vi "SPARC4_GUI.vi"() -> ()   [LabVIEW 2018]
uses:
  SPARC4_GUI/SPARC4_GUI.lvclass
  SPARC4_GUI/SPARC4_GUI.lvclass/SPARC4_GUI.ctl
  Channel GUI/Channel GUI.lvclass/Channel GUI.ctl
  Stream/Stream.lvclass/Stream.ctl
  Interface/Interface.lvclass/Interface.ctl
  Channel GUI/Channel GUI.lvclass
  Stream/Stream.lvclass
  State Machine/State Machine.lvclass
  Interface/Interface.lvclass
panel:
  out "Error":string
  in  "Tab Control 2":enum32{"Front Panel", "Setup Panel"}(tab)
  out "CCD Status":string
  out "Current image":string="CH1"
  out "% Acquired":u16
  out "Exposing":bool
  out "Temperature 2":i16
  out "Serial Number":u16
  out "Temperature Status":string
  in  "Base Name":string="IMG"
  in  "Exp Time 2":sgl=1e-05 min=1e-05
  in  "# Cubos":u32=1 min=1
  out "Exposições realizadas":u8(slide) max=2 scale=0.0..1.0
  in  "Acquire":bool
  in  "Command:":string
  out "Response:":string
  out "Initialization":bool
  in  "SEND":bool
  in  "IP Address:":string="//localhost"
  in  "Night Directory:":string="C:\\Users\\observer\\Desktop\\Imagens\\"
  in  "Stop Application":bool
  in  "Shutter Mode":u8(ring)=2 items=["Fully Auto", "OPEN", "CLOSED"]
  in  "Kinetic Series Length":u16=1 min=1
  in  "Cooler ON/OFF":u16(ring) items=["Cooler OFF", "Cooler ON"]
  in  "Temperature":i16=20 min=-80 max=20
  in  "Exposure Time":sgl=1e-05 min=1e-05
  in  "Readout Rate":u8(ring) items=["30 MHz", "20 MHz", "10 MHz", "  1 MHz"]
  in  "Pre-amp gain":u8(ring) items=["Gain 1", "Gain 2"]
  in  "EM Gain":u16=2
  in  "EM Mode":u8(ring) items=["Electron Multiplying", "Conventional"]
  in  "Sub Image":T1(radio)=enum."1024 x 1024"
  in  "Final Line":u16=1024
  in  "Final Column":u16=1024
  in  "Initial Cloumn":u16=1
  in  "Initial Line":u16=1
  in  "Binning":u16=1
  # "SPARC4 \nGeneral User Interface (GUI)"
  # "Command Acquisition Control"
  # "Channel 1: acquisition control & status"
  # "Temperature & Shutter"
  # "Timings"
  # "Horizontal pixel shift"
  # "EM Mode"
  # "Sub Image & Binning"
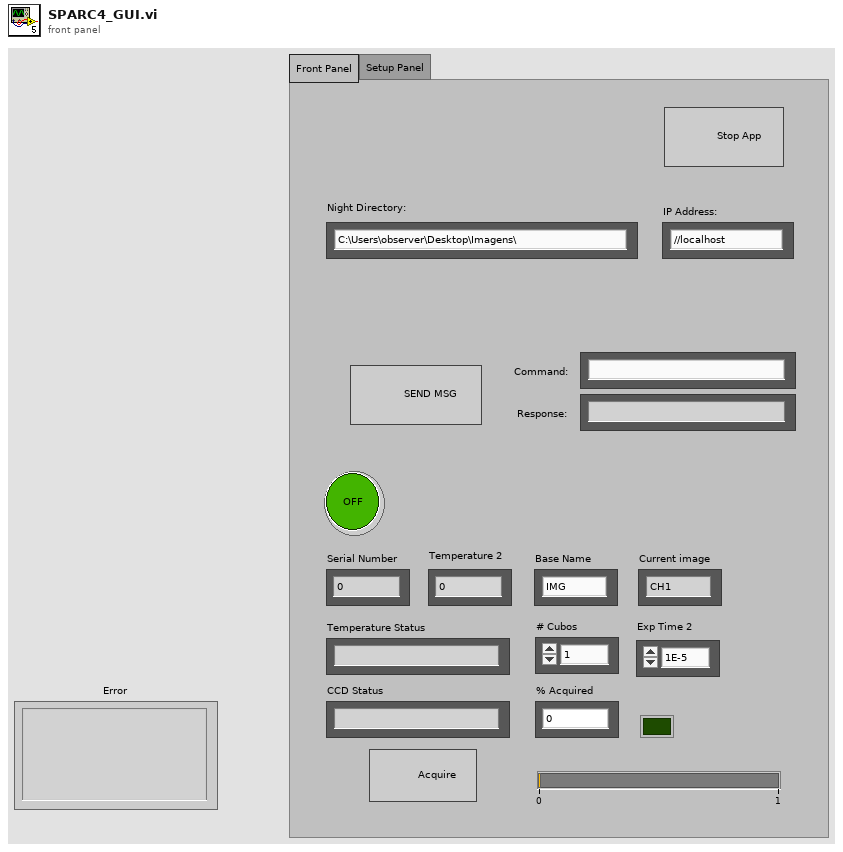
[diagram p1: front panel]
types:
  T1 = enum32{"256 x 256", "512 x 512", "1024 x 1024", "Custom"}
  T2 = cluster{"Exposure Time":sgl, "Pre-amp gain":u8, "Readout Rate":u8, "EM Mode":u8, "EM Gain":u16, "Binning":u16, "Initial Line":u16, "Initial Cloumn":u16, "Final Line":u16, "Final Column":u16, "Kinetic Series Length":u32, "Shutter Mode":u8, "Cooler ON/OFF":u16, "Temperature":i8, "Image Name":string, "Image Path":string, "# Images":u32}
  T3 = cluster{"% Acquired":u16, "Acquiring":bool, "Current image name":string, "Current sequence":u16, "CCD State":string}
  T4 = cluster{"Initialization":bool, "Serial Number":u16}
  T5 = cluster{"Current Temperature":i16, "Temperatue Status":string}
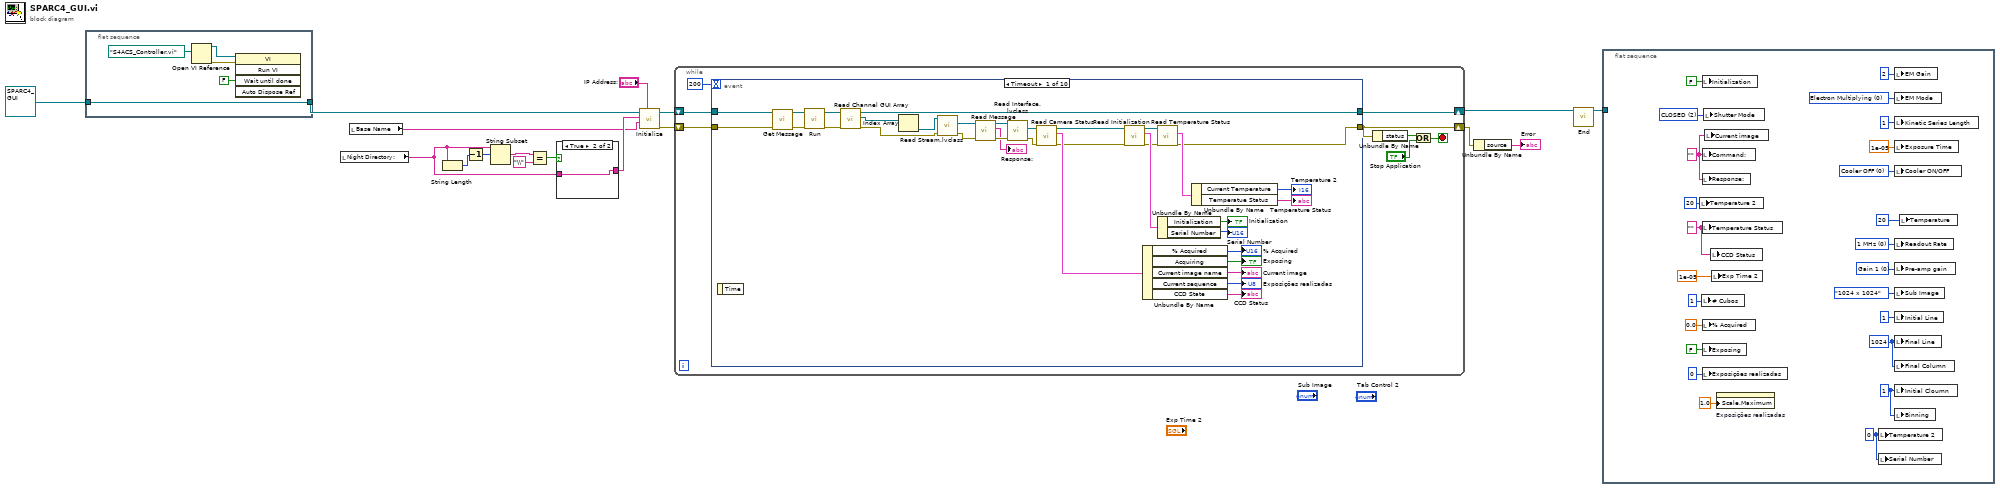
[diagram p0: block diagram]
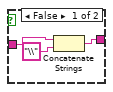
[diagram p2: hidden frame]
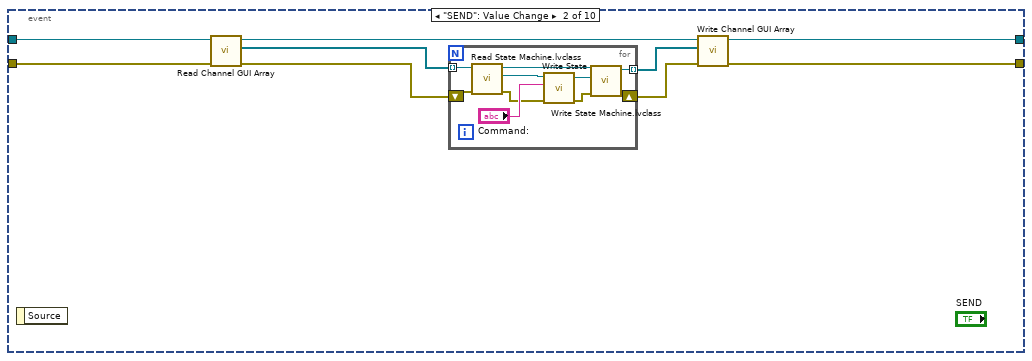
[diagram p3: hidden frame]
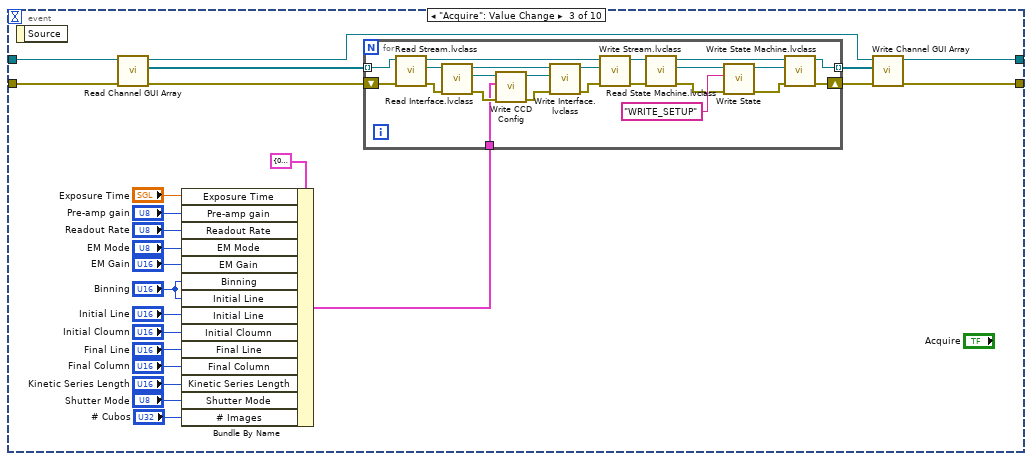
[diagram p4: hidden frame]
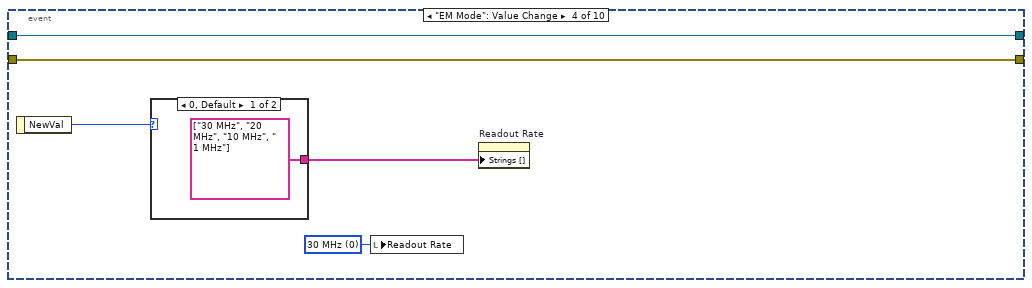
[diagram p5: hidden frame]
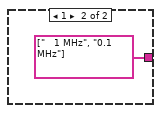
[diagram p6: hidden frame]
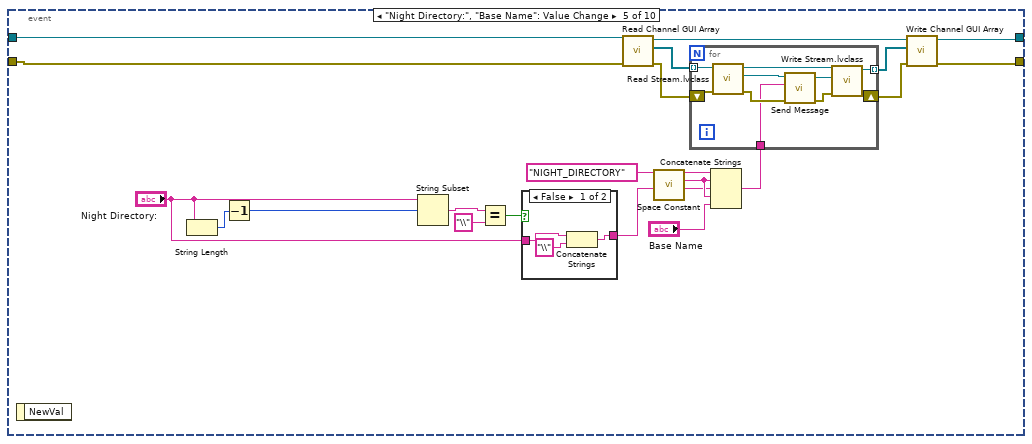
[diagram p7: hidden frame]
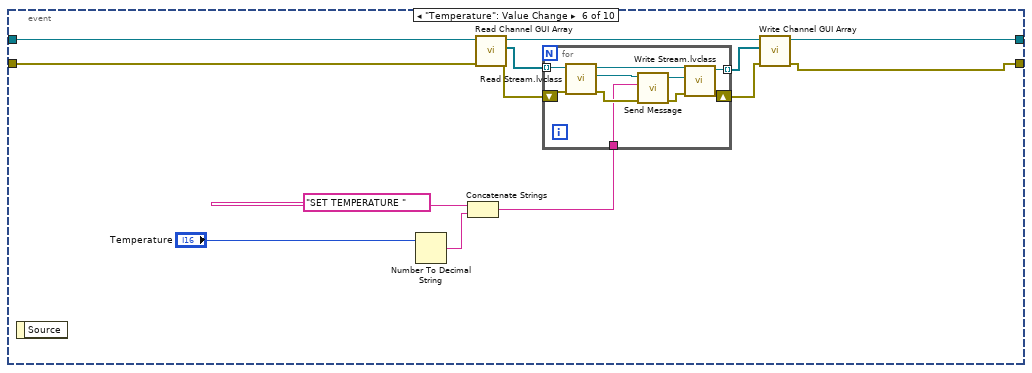
[diagram p9: hidden frame]
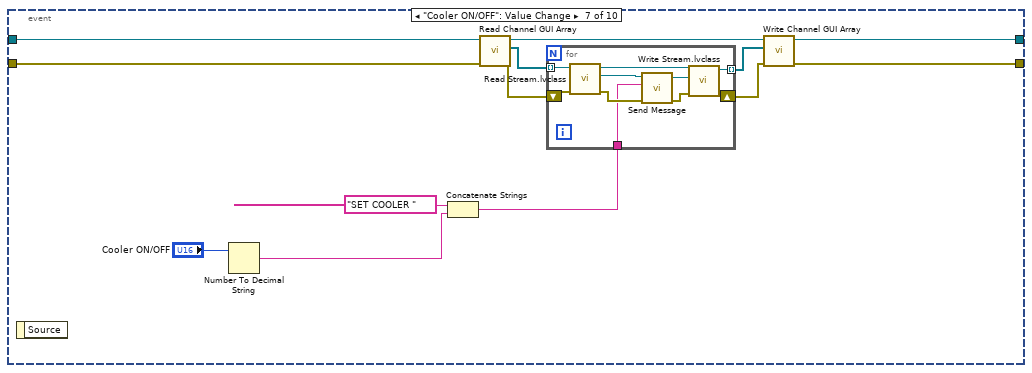
[diagram p10: hidden frame]
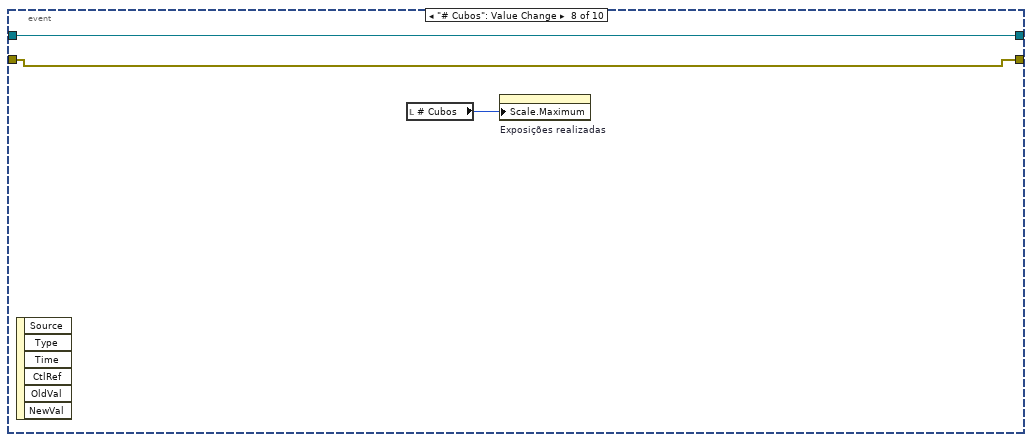
[diagram p11: hidden frame]
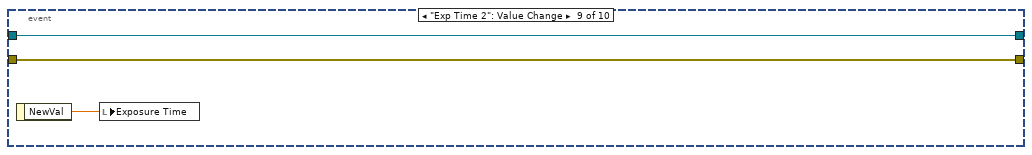
[diagram p12: hidden frame]
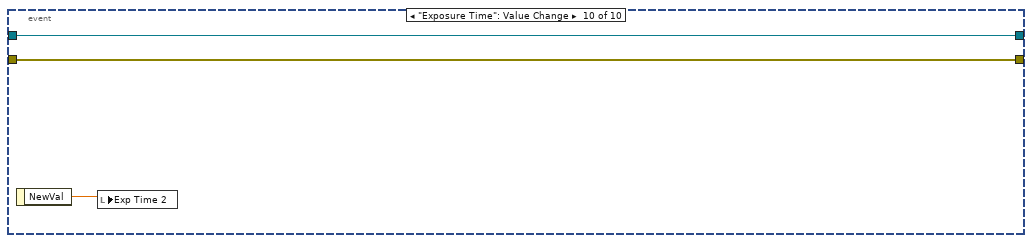
[diagram p13: hidden frame]
diagram:
  n1 = flat-sequence {
    tunnel: refnum<class "SPARC4_GUI.lvclass"> refnum ("SPARC4_GUI.lvclass") -> [w18]
    tunnel: [w18] -> w15
    frame #0 {
      n2 = Open VI Reference(vi path=path "S4ACS_Controller.vi") -> (vi reference=w22:refnum<vi>, error out=w21:errorcluster)  [unwired: 5 in]
      n3 = invoke class="VI" method="Run VI"(reference=w22, error in=w21, "Wait until done"=FALSE ("Wait Until Done")) -> ()  [unwired: 2 in, 5 out]
    }
  }
  n4 = local read "Night Directory:"() -> (w3:string)
  n5 = local read "Base Name"() -> (w1:string)
  n6 = String Length(string=w3) -> (length=w7:i32)
  n7 = Decrement(x=w7) -> (x-1=w6:i32)
  n8 = String Subset(string=w3, offset (0)=w6) -> (substring=w5:string)  [unwired: 1 in]
  n9 = Equal?(x=w5, y="\\") -> (x = y?=w4:bool)
  n10 = case shown="True" w4 {
    tunnel: [w25 w26] -> w2
    tunnel: w3 -> [w23 w26]
    frame False {
      n11 = Concatenate Strings(w23, "\\") -> (w25:string)
    }
    frame True {
    }
  }
  n12 = call "Initialize.vi"("IP"="IP Address:", "Image Name"=w1, "Night Directory:"=w2, "SPARC4_GUI in"=w15) -> ("error out"=w17:errorcluster, "SPARC4_GUI out"=w16:refnum<class "SPARC4_GUI.lvclass">)  [unwired: 6 in]
  n13 = while {
    shift-right: [w27] -> w10
    shift-left: w17 -> [w28]
    shift-right: [w30] -> w11
    shift-left: w16 -> [w29]
    stop <- w33 stop-if-true
    n14 = event shown="[0] Timeout" {
      selector: _ -> [_ _ _ _ _ _ _ _ _ _]
      dyn-events: _ -> [_ _ _ _ _ _ _ _ _ _]
      timeout: 200 -> [_ _ _ _ _ _ _ _ _ _]
      tunnel: w28 -> [w58 w76 w98 w138 w144 w178 w202 w223 w226 w229]
      tunnel: [w46 w69 w96 w138 w150 w184 w200 w223 w226 w229] -> w27
      tunnel: w29 -> [w59 w77 w99 w139 w143 w177 w203 w224 w227 w228]
      tunnel: [w57 w70 w97 w139 w151 w185 w201 w224 w227 w228] -> w30
      event Timeout {
        n15 = event-data() -> ()  [unwired: 1 in, 1 out]
        n16 = call "Get Message.vi"("error in (no error)"=w58, "SPARC4_GUI in"=w59) -> ("error out"=w61:errorcluster, "SPARC4_GUI out"=w60:refnum<class "SPARC4_GUI.lvclass">)  [unwired: 8 in]
        n17 = call "Run.vi"("error in (no error)"=w61, "SPARC4_GUI in"=w60) -> ("error out"=w66:errorcluster, "SPARC4_GUI out"=w65:refnum<class "SPARC4_GUI.lvclass">)  [unwired: 8 in]
        n18 = call "Read Channel GUI Array.vi"("error in (no error)"=w66, "SPARC4_GUI in"=w65) -> ("error out"=w36:errorcluster, "Channel GUI Array"=w38:refnum<class "Channel GUI.lvclass">[], "SPARC4_GUI out"=w57:refnum<class "SPARC4_GUI.lvclass">)  [unwired: 7 in]
        n19 = Index Array(array=w38) -> (element=w37:refnum<class "Channel GUI.lvclass">)  [unwired: 1 in]
        n20 = call "Read Stream.lvclass.vi"("error in (no error)"=w36, "Channel GUI in"=w37) -> ("error out"=w35:errorcluster, "Stream.lvclass"=w39:refnum<class "Stream.lvclass">)  [unwired: 7 in, 1 out]
        n21 = call "Read Message.vi"("error in (no error)"=w35, "Stream in"=w39) -> ("error out"=w44:errorcluster, "Message"=→"Response:":string, "Stream out"=w45:refnum<class "Stream.lvclass">)  [unwired: 7 in]
        n22 = call "Read Interface.lvclass.vi"("error in (no error)"=w44, "Stream in"=w45) -> ("error out"=w63:errorcluster, "Interface.lvclass"=w64:refnum<class "Interface.lvclass">)  [unwired: 7 in, 1 out]
        n23 = call "Read Camera Status.vi"("error in (no error)"=w63, "Interface in"=w64) -> ("error out"=w56:errorcluster, "Camera Status"=w62:T3, "Interface out"=w55:refnum<class "Interface.lvclass">)  [unwired: 7 in]
        n24 = call "Read Initialization.vi"("error in (no error)"=w56, "Interface in"=w55) -> ("error out"=w51:errorcluster, "Initialization"=w54:T4, "Interface out"=w50:refnum<class "Interface.lvclass">)  [unwired: 7 in]
        n25 = Unbundle By Name(w62) -> ("% Acquired"=→"% Acquired":u16, "Acquiring"=→"Exposing":bool, "Current image name"=→"Current image":string, "Current sequence"=→"Exposições realizadas":u16, "CCD State"=→"CCD Status":string)
        n26 = call "Read Temperature Status.vi"("error in (no error)"=w51, "Interface in"=w50) -> ("error out"=w46:errorcluster, "Temperature Status"=w49:T5)  [unwired: 7 in, 1 out]
        n27 = Unbundle By Name(w54) -> ("Initialization"=→"Initialization":bool, "Serial Number"=→"Serial Number":u16)
        n28 = Unbundle By Name(w49) -> ("Current Temperature"=→"Temperature 2":i16, "Temperatue Status"=→"Temperature Status":string)
      }
      event "SEND": Value Change {
        n29 = event-data() -> ()  [unwired: 1 in, 1 out]
        n30 = call "Read Channel GUI Array.vi"("error in (no error)"=w76, "SPARC4_GUI in"=w77) -> ("error out"=w72:errorcluster, "Channel GUI Array"=w75:refnum<class "Channel GUI.lvclass">[], "SPARC4_GUI out"=w71:refnum<class "SPARC4_GUI.lvclass">)  [unwired: 7 in]
        n31 = for {
          tunnel: w75 -> [w85] mode=indexing
          tunnel: [w86] -> w74 mode=indexing
          shift-right: [w80] -> w73
          shift-left: w72 -> [w79]
          n32 = call "Read State Machine.lvclass.vi"("error in (no error)"=w79, "Channel GUI in"=w85) -> ("error out"=w82:errorcluster, "State Machine.lvclass"=w83:refnum<class "State Machine.lvclass">, "Channel GUI out"=w84:refnum<class "Channel GUI.lvclass">)  [unwired: 7 in]
          n33 = call-dynamic "Write State.vi"("error in (no error)"=w82, "State"="Command:", "State Machine in"=w83) -> ("error out"=w81:errorcluster, "State Machine out"=w78:refnum<class "State Machine.lvclass">)  [unwired: 7 in]
          n34 = call "Write State Machine.lvclass.vi"("error in (no error)"=w81, "State Machine.lvclass"=w78, "Channel GUI in"=w84) -> ("error out"=w80:errorcluster, "Channel GUI out"=w86:refnum<class "Channel GUI.lvclass">)  [unwired: 7 in]
        }
        n35 = call "Write Channel GUI Array.vi"("error in (no error)"=w73, "Channel GUI Array"=w74, "SPARC4_GUI in"=w71) -> ("error out"=w69:errorcluster, "SPARC4_GUI out"=w70:refnum<class "SPARC4_GUI.lvclass">)  [unwired: 7 in]
      }
      event "Acquire": Value Change {
        n36 = event-data() -> ()  [unwired: 1 in, 1 out]
        n37 = call "Read Channel GUI Array.vi"("error in (no error)"=w98, "SPARC4_GUI in"=w99) -> ("error out"=w91:errorcluster, "Channel GUI Array"=w92:refnum<class "Channel GUI.lvclass">[], "SPARC4_GUI out"=w88:refnum<class "SPARC4_GUI.lvclass">)  [unwired: 7 in]
        n38 = Bundle By Name(cluster=T2 {"Exposure Time"=0.0, "Pre-amp gain"=0, "Readout Rate"=0, "EM Mode"=0, "EM Gain"=2, "Binning"=1, "Initial Line"=1, "Initial Cloumn"=1, "Final Line"=1024, "Final Column"=1024, "Kinetic Series Length"=0, "Shutter Mode"=2, "Cooler ON/OFF"=0, "Temperature"=20, "Image Name"="", "Image Path"="", "# Images"=1} ("CCD Config"), "Exposure Time"="Exposure Time", "Pre-amp gain"="Pre-amp gain", "Readout Rate"="Readout Rate", "EM Mode"="EM Mode", "EM Gain"="EM Gain", "Binning"="Binning", "Initial Line"="Binning", "Initial Line"="Initial Line", "Initial Cloumn"="Initial Cloumn", "Final Line"="Final Line", "Final Column"="Final Column", "Kinetic Series Length"="Kinetic Series Length", "Shutter Mode"="Shutter Mode", "# Images"="# Cubos") -> (w111:T2)
        n39 = for {
          tunnel: w111 -> [w132]
          tunnel: w92 -> [w115] mode=indexing
          tunnel: [w113] -> w90 mode=indexing
          shift-right: [w112] -> w89
          shift-left: w91 -> [w114]
          n40 = call "Read Stream.lvclass.vi"("error in (no error)"=w114, "Channel GUI in"=w115) -> ("error out"=w126:errorcluster, "Stream.lvclass"=w127:refnum<class "Stream.lvclass">, "Channel GUI out"=w123:refnum<class "Channel GUI.lvclass">)  [unwired: 7 in]
          n41 = call "Read Interface.lvclass.vi"("error in (no error)"=w126, "Stream in"=w127) -> ("error out"=w133:errorcluster, "Interface.lvclass"=w134:refnum<class "Interface.lvclass">, "Stream out"=w131:refnum<class "Stream.lvclass">)  [unwired: 7 in]
          n42 = call "Write CCD Config.vi"("error in (no error)"=w133, "CCD Config"=w132, "Interface in"=w134) -> ("error out"=w129:errorcluster, "Interface out"=w128:refnum<class "Interface.lvclass">)  [unwired: 7 in]
          n43 = call "Write Interface.lvclass.vi"("error in (no error)"=w129, "Interface.lvclass"=w128, "Stream in"=w131) -> ("error out"=w125:errorcluster, "Stream out"=w124:refnum<class "Stream.lvclass">)  [unwired: 7 in]
          n44 = call "Write Stream.lvclass.vi"("error in (no error)"=w125, "Stream.lvclass"=w124, "Channel GUI in"=w123) -> ("error out"=w122:errorcluster, "Channel GUI out"=w121:refnum<class "Channel GUI.lvclass">)  [unwired: 7 in]
          n45 = call "Read State Machine.lvclass.vi"("error in (no error)"=w122, "Channel GUI in"=w121) -> ("error out"=w116:errorcluster, "State Machine.lvclass"=w119:refnum<class "State Machine.lvclass">, "Channel GUI out"=w120:refnum<class "Channel GUI.lvclass">)  [unwired: 7 in]
          n46 = call-dynamic "Write State.vi"("error in (no error)"=w116, "State"="WRITE_SETUP", "State Machine in"=w119) -> ("error out"=w117:errorcluster, "State Machine out"=w118:refnum<class "State Machine.lvclass">)  [unwired: 7 in]
          n47 = call "Write State Machine.lvclass.vi"("error in (no error)"=w117, "State Machine.lvclass"=w118, "Channel GUI in"=w120) -> ("error out"=w112:errorcluster, "Channel GUI out"=w113:refnum<class "Channel GUI.lvclass">)  [unwired: 7 in]
        }
        n48 = call "Write Channel GUI Array.vi"("error in (no error)"=w89, "Channel GUI Array"=w90, "SPARC4_GUI in"=w88) -> ("error out"=w96:errorcluster, "SPARC4_GUI out"=w97:refnum<class "SPARC4_GUI.lvclass">)  [unwired: 7 in]
      }
      event "EM Mode": Value Change {
        w135 = u8 0 items=["30 MHz", "20 MHz", "10 MHz", "1 MHz"] ("Readout Rate")
        n49 = event-data() -> ("NewVal"=w136:u8)  [unwired: 1 in]
        n50 = case shown="0, Default" w136 {
          tunnel: [string[] ["30 MHz", "20 MHz", "10 MHz", "  1 MHz"] string[] ["   1 MHz", "0.1 MHz"]] -> w137
          frame 0, Default {
          }
          frame 1 {
          }
        }
        n51 = local write "Readout Rate"(w135) -> ()
        n52 = property on="Readout Rate" class="Ring (strict)"("Strings []"=w137) -> ()  [unwired: 2 in, 2 out]
      }
      event "Night Directory:", "Base Name": Value Change {
        n53 = event-data() -> ()  [unwired: 1 in, 1 out]
        n54 = String Length(string="Night Directory:") -> (length=w154:i32)
        n55 = Decrement(x=w154) -> (x-1=w155:i32)
        n56 = String Subset(string="Night Directory:", offset (0)=w155) -> (substring=w156:string)  [unwired: 1 in]
        n57 = Equal?(x=w156, y="\\") -> (x = y?=w157:bool)
        n58 = case shown="False" w157 {
          tunnel: [w174 w175] -> w152
          tunnel: "Night Directory:" -> [w172 w175]
          frame False {
            n59 = Concatenate Strings(w172, "\\") -> (w174:string)
          }
          frame True {
          }
        }
        n60 = call "Read Channel GUI Array.vi"("error in (no error)"=w144, "SPARC4_GUI in"=w143) -> ("error out"=w145:errorcluster, "Channel GUI Array"=w148:refnum<class "Channel GUI.lvclass">[], "SPARC4_GUI out"=w149:refnum<class "SPARC4_GUI.lvclass">)  [unwired: 7 in]
        n61 = call <vilib>:"Space Constant.vi"() -> ("String"=w160:string)
        n62 = Concatenate Strings("NIGHT_DIRECTORY" ("Message"), w160, w152, w160, "Base Name") -> (w142:string)
        n63 = for {
          tunnel: w148 -> [w170] mode=indexing
          tunnel: [w171] -> w147 mode=indexing
          shift-right: [w165] -> w146
          shift-left: w145 -> [w164]
          tunnel: w142 -> [w162]
          n64 = call "Read Stream.lvclass.vi"("error in (no error)"=w164, "Channel GUI in"=w170) -> ("error out"=w167:errorcluster, "Stream.lvclass"=w168:refnum<class "Stream.lvclass">, "Channel GUI out"=w169:refnum<class "Channel GUI.lvclass">)  [unwired: 7 in]
          n65 = call "Send Message.vi"("error in (no error)"=w167, "Message"=w162, "Stream in"=w168) -> ("error out"=w166:errorcluster, "Stream out"=w163:refnum<class "Stream.lvclass">)  [unwired: 7 in]
          n66 = call "Write Stream.lvclass.vi"("error in (no error)"=w166, "Stream.lvclass"=w163, "Channel GUI in"=w169) -> ("error out"=w165:errorcluster, "Channel GUI out"=w171:refnum<class "Channel GUI.lvclass">)  [unwired: 7 in]
        }
        n67 = call "Write Channel GUI Array.vi"("error in (no error)"=w146, "Channel GUI Array"=w147, "SPARC4_GUI in"=w149) -> ("error out"=w150:errorcluster, "SPARC4_GUI out"=w151:refnum<class "SPARC4_GUI.lvclass">)  [unwired: 7 in]
      }
      event "Temperature": Value Change {
        n68 = event-data() -> ()  [unwired: 1 in, 1 out]
        n69 = Number To Decimal String(number="Temperature") -> (decimal integer string=w187:string)  [unwired: 1 in]
        n70 = Concatenate Strings("SET TEMPERATURE " ("Message"), w187) -> (w176:string)
        n71 = call "Read Channel GUI Array.vi"("error in (no error)"=w178, "SPARC4_GUI in"=w177) -> ("error out"=w179:errorcluster, "Channel GUI Array"=w180:refnum<class "Channel GUI.lvclass">[], "SPARC4_GUI out"=w181:refnum<class "SPARC4_GUI.lvclass">)  [unwired: 7 in]
        n72 = for {
          tunnel: w180 -> [w197] mode=indexing
          tunnel: [w198] -> w182 mode=indexing
          shift-right: [w192] -> w183
          shift-left: w179 -> [w191]
          tunnel: w176 -> [w189]
          n73 = call "Read Stream.lvclass.vi"("error in (no error)"=w191, "Channel GUI in"=w197) -> ("error out"=w194:errorcluster, "Stream.lvclass"=w195:refnum<class "Stream.lvclass">, "Channel GUI out"=w196:refnum<class "Channel GUI.lvclass">)  [unwired: 7 in]
          n74 = call "Send Message.vi"("error in (no error)"=w194, "Message"=w189, "Stream in"=w195) -> ("error out"=w193:errorcluster, "Stream out"=w190:refnum<class "Stream.lvclass">)  [unwired: 7 in]
          n75 = call "Write Stream.lvclass.vi"("error in (no error)"=w193, "Stream.lvclass"=w190, "Channel GUI in"=w196) -> ("error out"=w192:errorcluster, "Channel GUI out"=w198:refnum<class "Channel GUI.lvclass">)  [unwired: 7 in]
        }
        n76 = call "Write Channel GUI Array.vi"("error in (no error)"=w183, "Channel GUI Array"=w182, "SPARC4_GUI in"=w181) -> ("error out"=w184:errorcluster, "SPARC4_GUI out"=w185:refnum<class "SPARC4_GUI.lvclass">)  [unwired: 7 in]
      }
      event "Cooler ON/OFF": Value Change {
        n77 = event-data() -> ()  [unwired: 1 in, 1 out]
        n78 = Number To Decimal String(number="Cooler ON/OFF") -> (decimal integer string=w209:string)  [unwired: 1 in]
        n79 = Concatenate Strings("SET COOLER ", w209) -> (w199:string)
        n80 = call "Read Channel GUI Array.vi"("error in (no error)"=w202, "SPARC4_GUI in"=w203) -> ("error out"=w204:errorcluster, "Channel GUI Array"=w205:refnum<class "Channel GUI.lvclass">[], "SPARC4_GUI out"=w206:refnum<class "SPARC4_GUI.lvclass">)  [unwired: 7 in]
        n81 = for {
          tunnel: w205 -> [w220] mode=indexing
          tunnel: [w221] -> w207 mode=indexing
          shift-right: [w215] -> w208
          shift-left: w204 -> [w214]
          tunnel: w199 -> [w212]
          n82 = call "Read Stream.lvclass.vi"("error in (no error)"=w214, "Channel GUI in"=w220) -> ("error out"=w217:errorcluster, "Stream.lvclass"=w218:refnum<class "Stream.lvclass">, "Channel GUI out"=w219:refnum<class "Channel GUI.lvclass">)  [unwired: 7 in]
          n83 = call "Send Message.vi"("error in (no error)"=w217, "Message"=w212, "Stream in"=w218) -> ("error out"=w216:errorcluster, "Stream out"=w213:refnum<class "Stream.lvclass">)  [unwired: 7 in]
          n84 = call "Write Stream.lvclass.vi"("error in (no error)"=w216, "Stream.lvclass"=w213, "Channel GUI in"=w219) -> ("error out"=w215:errorcluster, "Channel GUI out"=w221:refnum<class "Channel GUI.lvclass">)  [unwired: 7 in]
        }
        n85 = call "Write Channel GUI Array.vi"("error in (no error)"=w208, "Channel GUI Array"=w207, "SPARC4_GUI in"=w206) -> ("error out"=w200:errorcluster, "SPARC4_GUI out"=w201:refnum<class "SPARC4_GUI.lvclass">)  [unwired: 7 in]
      }
      event "# Cubos": Value Change {
        n86 = event-data() -> ()  [unwired: 1 in, 6 out]
        n87 = local read "# Cubos"() -> (w222:u32)
        n88 = property on="Exposições realizadas" class="Slide (strict)"("Scale.Maximum"=w222) -> ()  [unwired: 2 in, 2 out]
      }
      event "Exp Time 2": Value Change {
        n89 = event-data() -> ("NewVal"=w225:sgl)  [unwired: 1 in]
        n90 = local write "Exposure Time"(w225) -> ()
      }
      event "Exposure Time": Value Change {
        n91 = event-data() -> ("NewVal"=w230:sgl)  [unwired: 1 in]
        n92 = local write "Exp Time 2"(w230) -> ()
      }
    }
    n93 = Unbundle By Name(w27) -> ("status"=w32:bool)
    n94 = Or(x=w32, y="Stop Application") -> (x .or. y?=w33:bool)
  }
  n95 = Unbundle By Name(w10) -> ("source"=→"Error":string)
  n96 = call "End.vi"("SPARC4_GUI in"=w11) -> ("SPARC4_GUI out"=w12:refnum<class "SPARC4_GUI.lvclass">)  [unwired: 9 in, 1 out]
  n97 = flat-sequence {
    tunnel: w12 -> [_]
    frame #0 {
      w231 = i16 0 ("Temperature 2")
      w235 = u8 2 items=["Fully Auto", "OPEN", "CLOSED"] ("Shutter Mode")
      w232 = "" ("Command:")
      w237 = u16 1024 ("Final Line")
      w236 = u16 1 ("Initial Cloumn")
      w240 = u8 0 items=["Gain 1", "Gain 2"] ("Pre-amp gain")
      w241 = u8 0 items=["1 MHz", "10 MHz", "20 MHz", "30 MHz"] ("Readout Rate")
      w243 = u16 0 items=["Cooler OFF", "Cooler ON"] ("Cooler ON/OFF")
      w246 = u8 0 items=["Electron Multiplying", "Conventional"] ("EM Mode")
      w233 = "" ("Temperature Status")
      n98 = local write "Temperature 2"(20 ("Temperature")) -> ()
      n99 = local write "# Cubos"(u32 1 ("# Ciclos")) -> ()
      n100 = local write "Initialization"(FALSE ("Initialization")) -> ()
      n101 = local write "Command:"(w232) -> ()
      n102 = local write "Response:"(w232) -> ()
      n103 = local write "Temperature Status"(w233) -> ()
      n104 = local write "% Acquired"(0.0 ("% Acquired")) -> ()
      n105 = local write "Exposing"(FALSE ("Exposing")) -> ()
      n106 = local write "Exposições realizadas"(u8 0 ("Exposições realizadas")) -> ()
      n107 = local write "Shutter Mode"(w235) -> ()
      n108 = local write "Current image"(w232) -> ()
      n109 = local write "CCD Status"(w233) -> ()
      n110 = local write "Exp Time 2"(1e-05 ("Exposure Time 2")) -> ()
      n111 = property on="Exposições realizadas" class="Slide (strict)"("Scale.Maximum"=1.0 ("Scale.Range:Maximum")) -> ()  [unwired: 2 in, 2 out]
      n112 = local write "Temperature 2"(w231) -> ()
      n113 = local write "Serial Number"(w231) -> ()
      n114 = local write "EM Gain"(u16 2 ("EM Gain")) -> ()
      n115 = local write "EM Mode"(w246) -> ()
      n116 = local write "Kinetic Series Length"(u16 1 ("Kinetic Series Length")) -> ()
      n117 = local write "Exposure Time"(1e-05 ("Exposure Time")) -> ()
      n118 = local write "Cooler ON/OFF"(w243) -> ()
      n119 = local write "Readout Rate"(w241) -> ()
      n120 = local write "Pre-amp gain"(w240) -> ()
      n121 = local write "Sub Image"(T1."1024 x 1024" ("Sub Image")) -> ()
      n122 = local write "Initial Line"(u16 1 ("Initial Line")) -> ()
      n123 = local write "Final Line"(w237) -> ()
      n124 = local write "Final Column"(w237) -> ()
      n125 = local write "Initial Cloumn"(w236) -> ()
      n126 = local write "Binning"(w236) -> ()
      n127 = local write "Temperature"(i16 20 ("Set temperature")) -> ()
    }
  }
